vi "Load Robot Program.vi"(8 "error in (no error)":errorcluster, 10 "Program_Name":string, 11 "UR5 Robot in":refnum<class "UR5 Robot.lvclass">) -> (0 "error out":errorcluster, 3 "UR5 Robot out":refnum<class "UR5 Robot.lvclass">)   [LabVIEW 2018, in "UR5 Robot.lvlib" / "UR5 Robot.lvclass"]
uses:
  UR5 Robot.lvclass
  UR5 Robot.lvclass/UR5 Robot.ctl
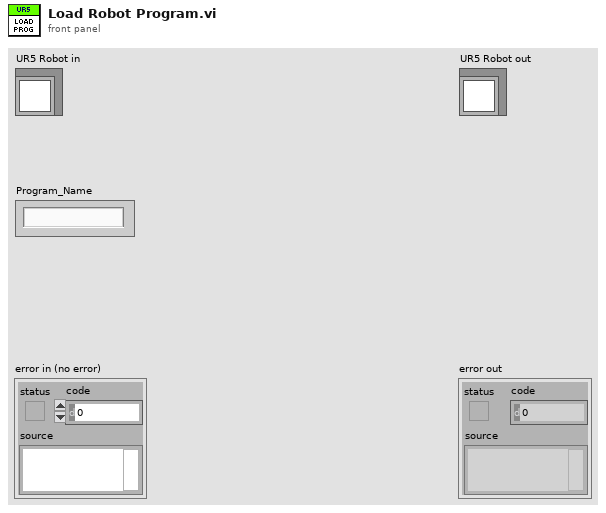
[diagram p1: front panel]
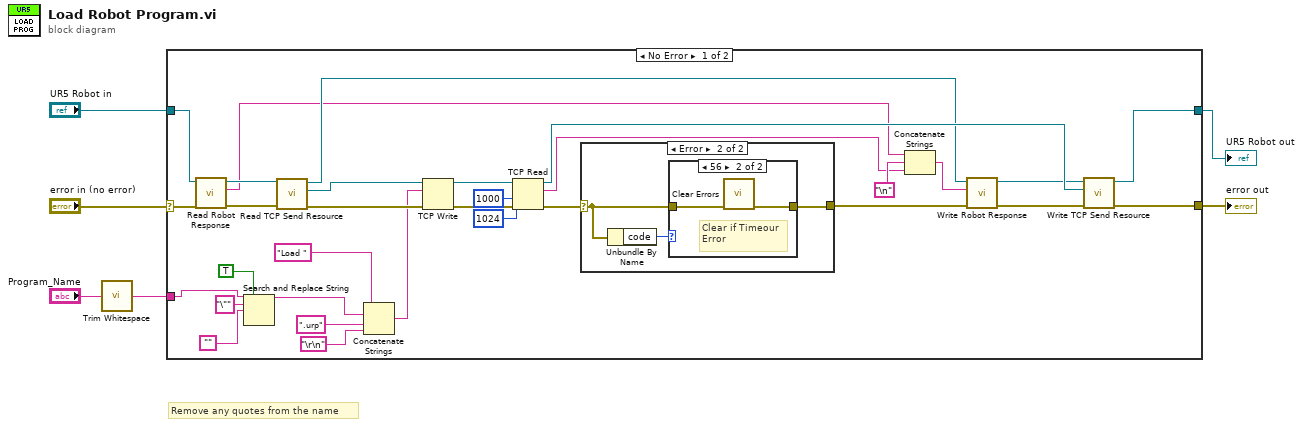
[diagram p0: block diagram]
diagram:
  # "Remove any quotes from the name"
  n1 = call <vilib>:"Trim Whitespace.vi"("string"="Program_Name") -> ("trimmed string"=w1:string)  [unwired: 1 in]
  n2 = case shown="No Error" "error in (no error)" {
    selector: "error in (no error)" -> [w24 w46]
    tunnel: [w27 w46] -> w5
    tunnel: [w25 w45] -> w4
    tunnel: "UR5 Robot in" -> [w22 w45]
    tunnel: w1 -> [w9 _]
    frame No Error {
      n3 = call "Read Robot Response.vi"("error in (no error)"=w24, "UR5 Robot in"=w22) -> ("error out"=w23:errorcluster, "Robot Response"=w16:string, "UR5 Robot out"=w21:refnum<class "UR5 Robot.lvclass">)  [unwired: 7 in]
      n4 = Search and Replace String(replace all?=TRUE ("replace all? (F)"), input string=w9, search string="\"", replace string="") -> (result string=w7:string)  [unwired: 4 in, 3 out]
      n5 = call "Read TCP Send Resource.vi"("error in (no error)"=w23, "UR5 Robot in"=w21) -> ("error out"=w31:errorcluster, "TCP Send Resource"=w32:refnum<k5>, "UR5 Robot out"=w18:refnum<class "UR5 Robot.lvclass">)  [unwired: 7 in]
      n6 = Concatenate Strings("Load ", w7, ".urp" ("string"), "\r\n") -> (w28:string)
      n7 = TCP Write(connection ID=w32, data in=w28, error in (no error)=w31) -> (connection ID out=w36:refnum<k5>, error out=w35:errorcluster)  [unwired: 1 in, 1 out]
      n8 = TCP Read(connection ID=w36, bytes to read=1024, error in (no error)=w35, 9:1000 ("timeout ms (25000)")) -> (connection ID out=w26:refnum<k5>, data out=w14:string, error out=w37:errorcluster)  [unwired: 1 in]
      n9 = case shown="Error" w37 {
        selector: w37 -> [w38 w40]
        tunnel: [w38 w39] -> w20
        frame No Error {
        }
        frame Error {
          n10 = Unbundle By Name(w40) -> ("code"=w41:i32)
          n11 = case shown="56" w41 {
            tunnel: w40 -> [w42 w44]
            tunnel: [w42 w43] -> w39
            frame 0, Default {
            }
            frame 56 {
              # "Clear if Timeour\nError"
              n12 = call <vilib>:"Clear Errors.vi"("error in (no error)"=w44) -> ("error out"=w43:errorcluster)  [unwired: 5 in, 1 out]
            }
          }
        }
      }
      n13 = Concatenate Strings(w16, "\n", w14) -> (w13:string)
      n14 = call "Write Robot Response.vi"("error in (no error)"=w20, "Robot Response"=w13, "UR5 Robot in"=w18) -> ("error out"=w19:errorcluster, "UR5 Robot out"=w17:refnum<class "UR5 Robot.lvclass">)  [unwired: 7 in]
      n15 = call "Write TCP Send Resource.vi"("error in (no error)"=w19, "TCP Send Resource"=w26, "UR5 Robot in"=w17) -> ("error out"=w27:errorcluster, "UR5 Robot out"=w25:refnum<class "UR5 Robot.lvclass">)  [unwired: 7 in]
    }
    frame Error {
    }
  }
  "error out" <- w5
  "UR5 Robot out" <- w4
